vi "Enable Short.vi"(8 "error in (no error)":errorcluster, 10 "Enable Short (F: False)":bool, 11 "VISA resource name":refnum<visa-resource-name>) -> (0 "error out":errorcluster, 3 "VISA resource name out":refnum<visa-resource-name>)   [LabVIEW 2019, in "BK Precision 8500B Series.lvlib"]
doc: "Enables or disables shorting the input. When short is enabled, the load module will sink maximum current with the present operating range."
uses:
  <instrlib>/BK Precision 8500B Series/BK Precision 8500B Series.lvlib
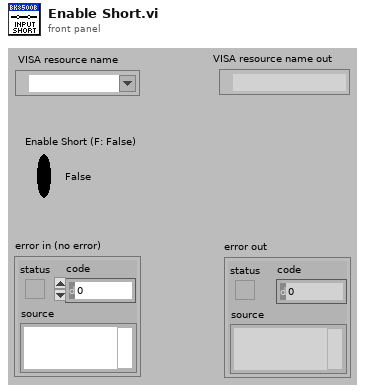
[diagram p1: front panel]
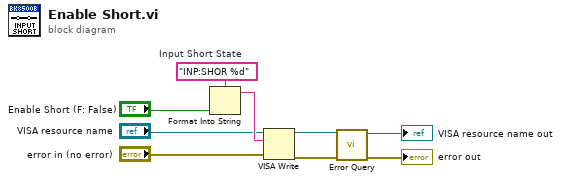
[diagram p0: block diagram]
diagram:
  w7 = "INP:SHOR %d"  # Input Short State
  n1 = Format Into String(format string=w7, "Enable Short (F: False)") -> (resulting string=w6:string)  [unwired: 2 in, 1 out]
  n2 = VISA Write(VISA resource name="VISA resource name", write buffer=w6, error in (no error)="error in (no error)") -> (VISA resource name out=w4:refnum<visa-resource-name>, error out=w3:errorcluster)  [unwired: 1 out]
  n3 = call <instrlib>:"Error Query.vi"("error in (no error)"=w3, "VISA resource name"=w4) -> ("error out"=→"error out":errorcluster, "VISA resource name out"=→"VISA resource name out":refnum<visa-resource-name>)  [unwired: 6 in, 2 out]
